vi "Profile.vi"() -> ()   [LabVIEW 2020]
panel:
  out "DBom":dbl
  out "DNatt":dbl
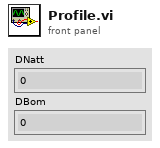
[diagram p1: front panel]
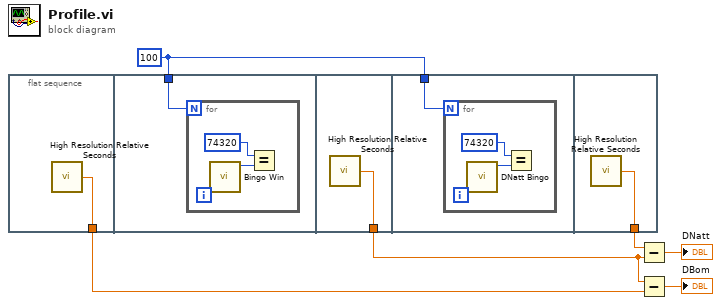
[diagram p0: block diagram]
diagram:
  w1 = 100
  n1 = flat-sequence {
    tunnel: [w7] -> w4
    tunnel: w1 -> [w8]
    tunnel: [w11] -> w5
    tunnel: w1 -> [w12]
    tunnel: [w15] -> w6
    frame #0 {
      n2 = call <vilib>:"High Resolution Relative Seconds.vi"() -> ("relative seconds"=w7:dbl)
    }
    frame #1 {
      n3 = for {
        N: w8 -> [_]
        n4 = call "Bingo Win.vi"() -> ("x*y"=w10:i32)  [unwired: 11 in]
        n5 = Equal?(x=74320 ("x*y"), y=w10) -> ()  [unwired: 1 out]
      }
    }
    frame #2 {
      n6 = call <vilib>:"High Resolution Relative Seconds.vi"() -> ("relative seconds"=w11:dbl)
    }
    frame #3 {
      n7 = for {
        N: w12 -> [_]
        n8 = call "DNatt Bingo.vi"() -> ("Answer"=w14:i32)  [unwired: 11 in]
        n9 = Equal?(x=74320 ("x*y"), y=w14) -> ()  [unwired: 1 out]
      }
    }
    frame #4 {
      n10 = call <vilib>:"High Resolution Relative Seconds.vi"() -> ("relative seconds"=w15:dbl)
    }
  }
  n11 = Subtract(x=w6, y=w5) -> (x-y=→"DNatt":dbl)
  n12 = Subtract(x=w5, y=w4) -> (x-y=→"DBom":dbl)
